vi "Array Investigation Part 3.vi"() -> ()   [LabVIEW 2014]
doc: "This VI is an exercise in the LabVIEW Core I course.\n\nEnter the number of columns and rows you want generated, then run the VI. This VI generates an array with the number of rows and columns you specify."
panel:
  out "Second Column":dbl[](array[numeric])
  out "Third Row":dbl[](array[numeric])
  out "Intensity Graph":dbl[][](graph)
  out "Array":dbl[][](array[numeric])
  in  "Rows":i32=80
  in  "Columns":i32=80
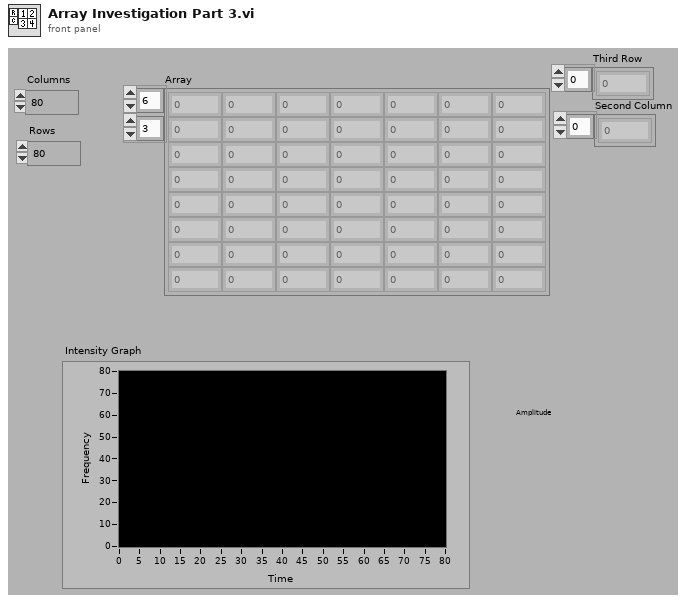
[diagram p1: front panel]
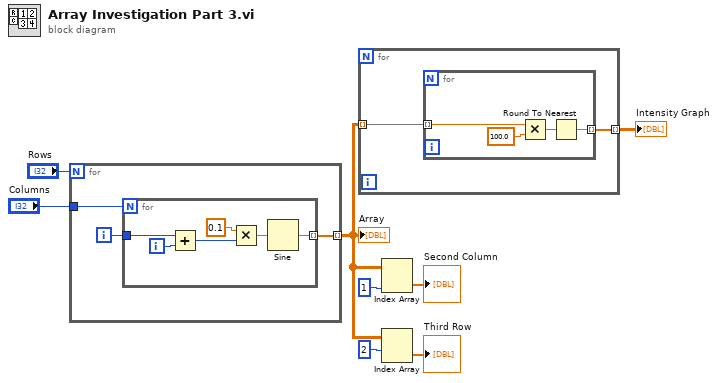
[diagram p0: block diagram]
diagram:
  n1 = for {
    N: "Rows" -> [_]
    tunnel: [w11] -> w3 mode=indexing
    tunnel: "Columns" -> [w10]
    i -> [w9]
    n2 = for {
      N: w10 -> [_]
      tunnel: [w17] -> w11 mode=indexing
      tunnel: w9 -> [w14]
      i -> [w15]
      n3 = Add(x=w14, y=w15) -> (x+y=w16:i32)
      n4 = Multiply(x=0.1, y=w16) -> (x*y=w13:dbl)
      n5 = Sine(x=w13) -> (sin(x)=w17:dbl)
    }
  }
  "Array" <- w3
  n6 = for {
    tunnel: w3 -> [w19] mode=indexing
    tunnel: [w18] -> w6 mode=indexing
    n7 = for {
      tunnel: w19 -> [w22] mode=indexing
      tunnel: [w20] -> w18 mode=indexing
      n8 = Multiply(x=w22, y=100.0) -> (x*y=w21:dbl)
      n9 = Round To Nearest(number=w21) -> (nearest integer value=w20:dbl)
    }
  }
  "Intensity Graph" <- w6
  n10 = Index Array(array=w3, index (col)=1 ("disabled index (col)")) -> (element=→"Second Column":dbl[])  [unwired: 1 in]
  n11 = Index Array(array=w3, index (row)=2) -> (element=→"Third Row":dbl[])  [unwired: 1 in]
